vi "PWV_BH(SubVI).vi"(10 "Diameter (mm)":dbl[](array[numeric]), 11 "Pressure (mmhg)":dbl[](array[numeric])) -> (0 "PWV (m/s) (BH Diastole)":dbl, 2 "PWV w/f (m/s) BH":dbl[](graph), 3 "PWV (m/s) (BH approx.)":dbl)   [LabVIEW 2017]
panel:
  out "XY Graph":cluster{"Mean Distal Diameter":dbl[], "Y":dbl[]}(graph)
  out "Waveform Graph 3":dbl[](graph)
  out "Waveform Graph 2":dbl[][](graph)
  out "Waveform Graph":dbl[][](graph)
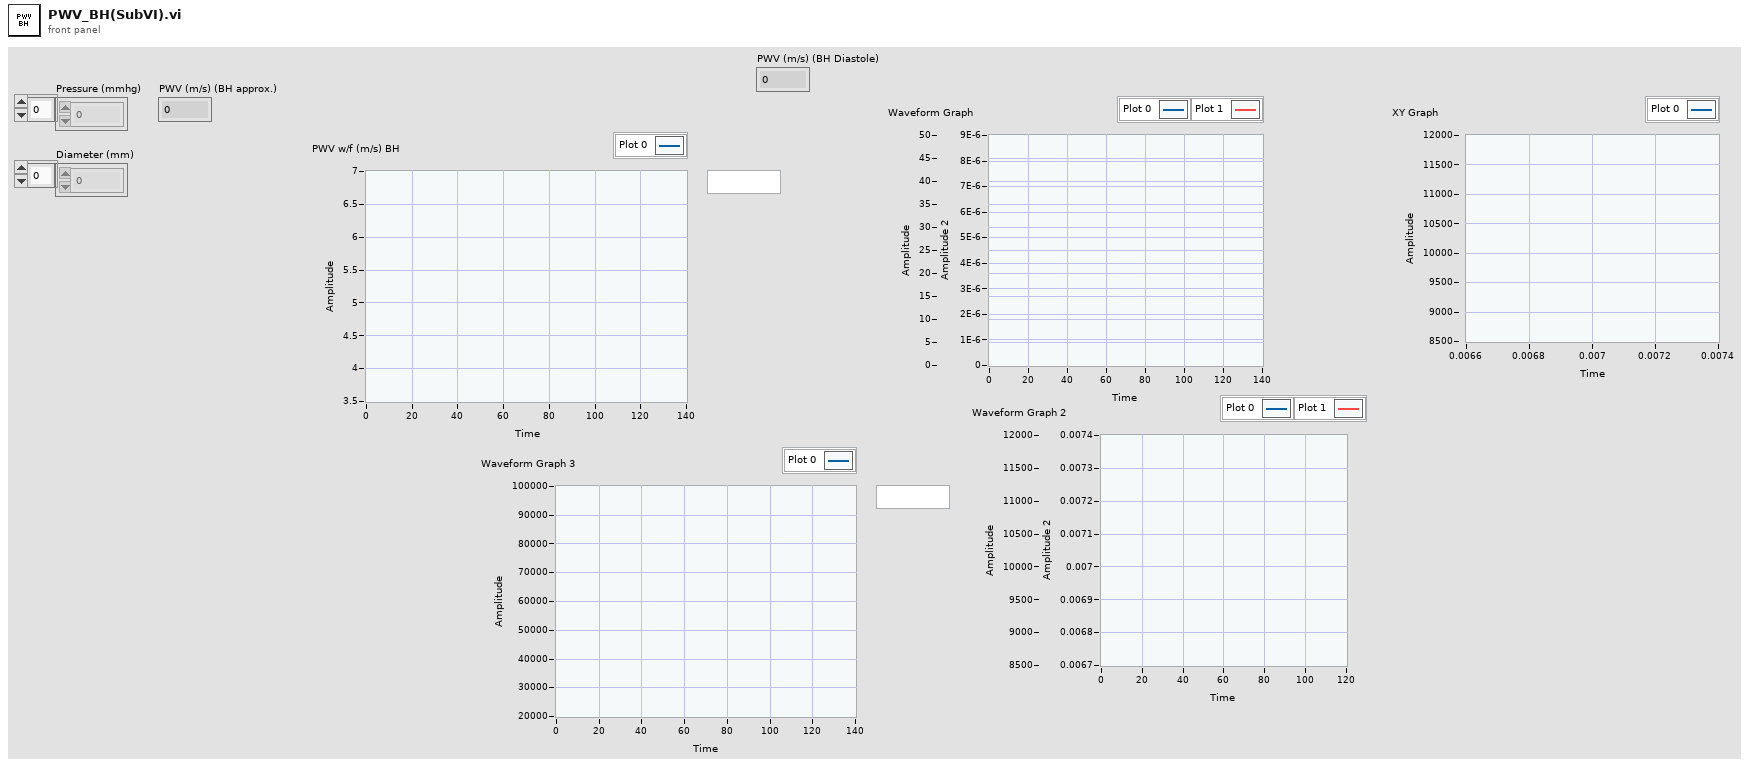
[diagram p1: front panel]
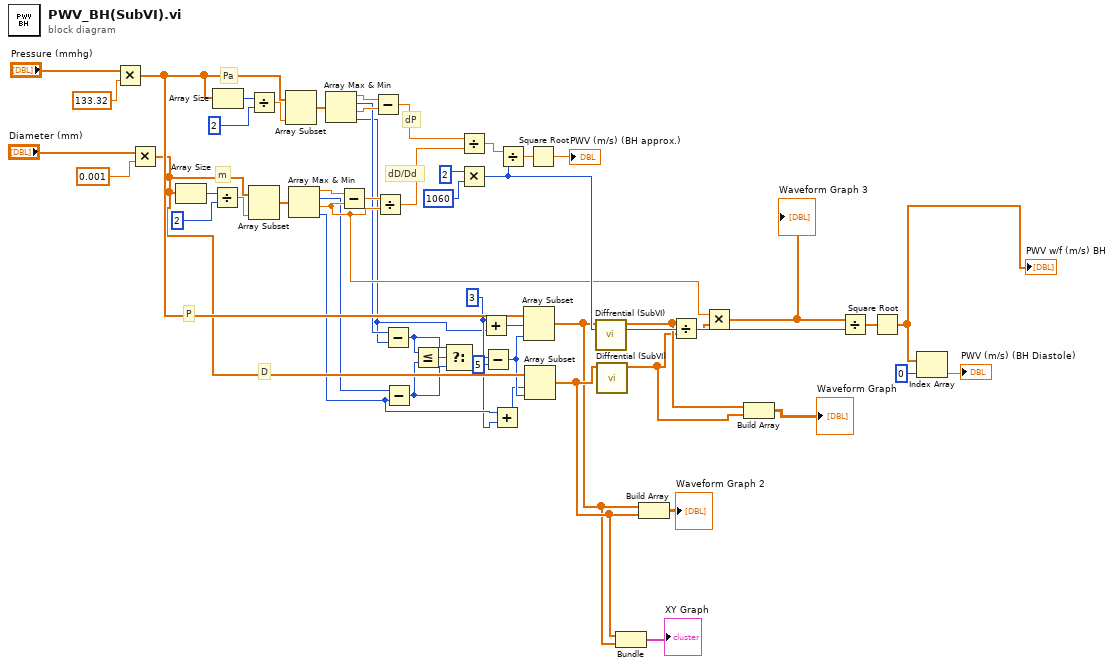
[diagram p0: block diagram]
diagram:
  w6 = 3 ("y")
  # "D"
  # "P"
  # "dD/Dd"
  # "dP"
  # "m"
  # "Pa"
  n1 = Multiply(x="Pressure (mmhg)", y=133.32 ("x")) -> (x*y=w24:dbl[])
  n2 = Multiply(x="Diameter (mm)", y=0.001 ("x")) -> (x*y=w23:dbl[])
  n3 = Array Size(array=w23) -> (size(s)=w35:i32)
  n4 = Divide(x=w35, y=2) -> (x/y=w33:dbl)
  n5 = Array Size(array=w24) -> (size(s)=w28:i32)
  n6 = Divide(x=w28, y=2) -> (x/y=w30:dbl)
  n7 = Array Subset(array=w23, length=w33) -> (w32:dbl[])  [unwired: 1 in]
  n8 = Array Subset(array=w24, length=w30) -> (w31:dbl[])  [unwired: 1 in]
  n9 = Array Max & Min(array=w32) -> (max value=w41:dbl, max index (indices)=w22:i32, min value=w51:dbl, min index (indices)=w7:i32)
  n10 = Array Max & Min(array=w31) -> (max value=w40:dbl, max index (indices)=w9:i32, min value=w42:dbl, min index (indices)=w4:i32)
  n11 = Subtract(x=w41, y=w51) -> (x-y=w43:dbl)
  n12 = Subtract(x=w40, y=w42) -> (x-y=w44:dbl)
  n13 = Divide(x=w43, y=w51) -> (x/y=w45:dbl)
  n14 = Subtract(x=w9, y=w4) -> (x-y=w19:i32)
  n15 = Subtract(x=w22, y=w7) -> (x-y=w18:i32)
  n16 = Less Or Equal?(x=w19, y=w18) -> (x <= y?=w20:bool)
  n17 = Select(t=w19, s=w20, f=w18) -> (s? t:f=w12:i32)
  n18 = Divide(x=w44, y=w45) -> (x/y=w46:dbl)
  n19 = Multiply(x=2, y=1060) -> (x*y=w52:i32)
  n20 = Add(x=w6, y=w4) -> (x+y=w8:i32)
  n21 = Subtract(x=w12, y=5) -> (x-y=w10:i32)
  n22 = Add(x=w7, y=w6) -> (x+y=w5:i32)
  n23 = Divide(x=w46, y=w52) -> (x/y=w49:dbl)
  n24 = Array Subset(array=w24, index=w8, length=w10) -> (w1:dbl[])
  n25 = Array Subset(array=w23, index=w5, length=w10) -> (w2:dbl[])
  n26 = Square Root(x=w49) -> (sqrt(x)=→"PWV (m/s) (BH approx.)":dbl)
  n27 = call "Diffrential (SubVI).vi"("d(n)"=w1) -> ("d(n)-d(n+1)"=w15:dbl[])  [unwired: 10 in]
  n28 = call "Diffrential (SubVI).vi"("d(n)"=w2) -> ("d(n)-d(n+1)"=w14:dbl[])  [unwired: 10 in]
  n29 = Bundle(w2, w1) -> (→"XY Graph":cluster{dbl[], dbl[]})  [unwired: 1 in]
  n30 = Build Array(w1, w2) -> (→"Waveform Graph 2":dbl[][])
  n31 = Divide(x=w15, y=w14) -> (x/y=w25:dbl[])
  n32 = Multiply(x=w51, y=w25) -> (x*y=w16:dbl[])
  "Waveform Graph 3" <- w16
  n33 = Build Array(w15, w14) -> (→"Waveform Graph":dbl[][])
  n34 = Divide(x=w16, y=w52) -> (x/y=w53:dbl[])
  n35 = Square Root(x=w53) -> (sqrt(x)=w21:dbl[])
  "PWV w/f (m/s) BH" <- w21
  n36 = Index Array(array=w21, index=0) -> (element=→"PWV (m/s) (BH Diastole)":dbl)
